vi "Create License.vi"() -> ()   [LabVIEW 2013]
panel:
  out "error out":errorcluster caption="错误输出"
  in  "错误输入":errorcluster
  out "MD5 message-digest":string caption="License"
  in  "CPU ID":string
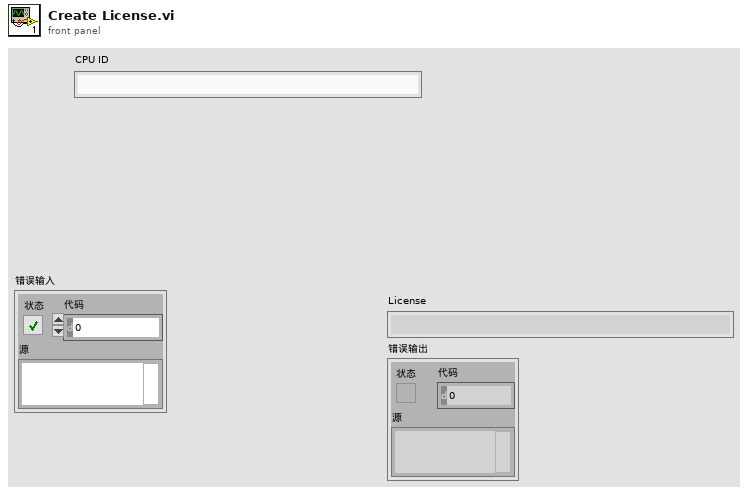
[diagram p1: front panel]
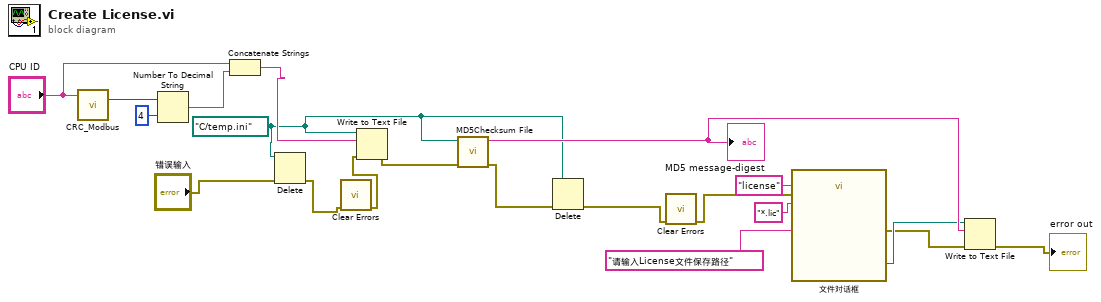
[diagram p0: block diagram]
diagram:
  w12 = path "C:/temp.ini" ("文件（使用对话框）")
  n1 = call "CRC_Modbus.vi"("字符串"="CPU ID") -> ("输出变量"=w20:u16)  [unwired: 10 in]
  n2 = Number To Decimal String(number=w20, width (-)=i16 4 ("宽度(-)")) -> (decimal integer string=w18:string)
  n3 = Concatenate Strings("CPU ID", w18) -> (w17:string)
  n4 = Delete(path (use dialog)=w12, error in="错误输入") -> (error out=w6:errorcluster)  [unwired: 3 in, 2 out]
  n5 = call <vilib>:"Clear Errors.vi"("error in (no error)"=w6) -> ("error out"=w5:errorcluster)  [unwired: 6 in]
  n6 = Write to Text File(file (use dialog)=w12, text=w17, error in=w5) -> (error out=w16:errorcluster)  [unwired: 1 in, 2 out]
  n7 = call <vilib>:"MD5Checksum File.vi"("error in (no error)"=w16, "Path"=w12) -> ("error out"=w13:errorcluster, "MD5 message-digest"=w15:string)  [unwired: 8 in]
  "MD5 message-digest" <- w15
  n8 = Delete(path (use dialog)=w12, error in=w13) -> (error out=w8:errorcluster)  [unwired: 3 in, 2 out]
  n9 = call <vilib>:"Clear Errors.vi"("error in (no error)"=w8) -> ("error out"=w7:errorcluster)  [unwired: 6 in]
  n10 = call "文件对话框"("prompt"="请输入License文件保存路径", "default name"="license", "error in"=w7, "pattern (all files)"="*.lic" ("pattern label")) -> ("selected path"=w14:path, "error out"=w10:errorcluster)  [unwired: 8 in, 2 out]
  n11 = Write to Text File(file (use dialog)=w14, text=w15, error in=w10) -> (error out=→"error out":errorcluster)  [unwired: 1 in, 2 out]
